vi "Get Valid String.vi"(10 "String":string, 11 "DBL":dbl format="%_11f") -> (2 "F-format string":string, 3 "number":dbl format="%#.6f")   [LabVIEW 2021]
doc: "get valid pricesion of Num or String.\n2016-08-31 11:45:50\n蒋松\nsina：@sushu1051"
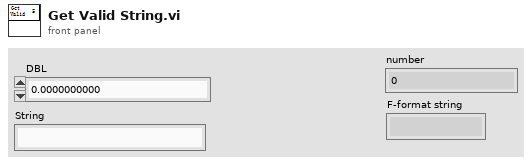
[diagram p1: front panel]
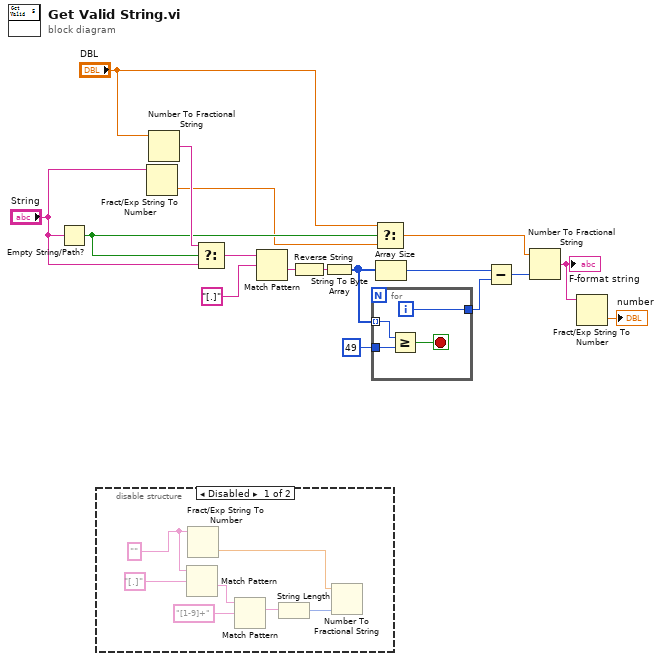
[diagram p0: block diagram]
diagram:
  n1 = Empty String/Path?(string/path="String") -> (empty?=w11:bool)
  n2 = disable-structure shown="Disabled" {
    frame Disabled {
      w18 = "" ("String")
      n3 = Match Pattern(string=w18, regular expression="[.]") -> (after substring=w23:string)  [unwired: 1 in, 3 out]
      n4 = Fract/Exp String To Number(string=w18) -> (number=w20:dbl)  [unwired: 3 in, 1 out]
      n5 = Match Pattern(string=w23, regular expression="[1-9]+") -> (match substring=w24:string)  [unwired: 1 in, 3 out]
      n6 = String Length(string=w24) -> (length=w19:i32)
      n7 = Number To Fractional String(number=w20, precision (6)=w19) -> ()  [unwired: 2 in, 1 out]
    }
    frame Enabled {
    }
  }
  n8 = Fract/Exp String To Number(string="String") -> (number=w8:dbl)  [unwired: 3 in, 1 out]
  n9 = Number To Fractional String(number="DBL") -> (F-format string=w14:string)  [unwired: 3 in]
  n10 = Select(t=w14, s=w11, f="String") -> (s? t:f=w13:string)
  n11 = Match Pattern(string=w13, regular expression="[.]") -> (after substring=w7:string)  [unwired: 1 in, 3 out]
  n12 = Reverse String(1:w7) -> (0:w6:string)
  n13 = String To Byte Array(string=w6) -> (unsigned byte array=w4:u8[])
  n14 = for {
    tunnel: w4 -> [w28] mode=indexing
    tunnel: u8 49 ("y") -> [w27]
    tunnel: [w25] -> w2
    i -> [w25]
    stop <- w26 stop-if-true
    n15 = Greater Or Equal?(x=w28, y=w27) -> (x >= y?=w26:bool)
  }
  n16 = Select(t="DBL", s=w11, f=w8) -> (s? t:f=w9:dbl)
  n17 = Array Size(array=w4) -> (size(s)=w3:i32)
  n18 = Subtract(x=w3, y=w2) -> (x-y=w1:i32)
  n19 = Number To Fractional String(number=w9, precision (6)=w1) -> (F-format string=w16:string)  [unwired: 2 in]
  "F-format string" <- w16
  n20 = Fract/Exp String To Number(string=w16) -> (number=→"number":dbl)  [unwired: 3 in, 1 out]
